vi "S2C_5190CR_Proc_Globals.vi"() -> ()   [LabVIEW 2015]
doc: "Globals for the 5190CR process."
panel:
  out "5190-Tcp":refnum<k5>
  out "5190-Refs":string[][](array[string])
  in  "5190-VI":refnum<vi>
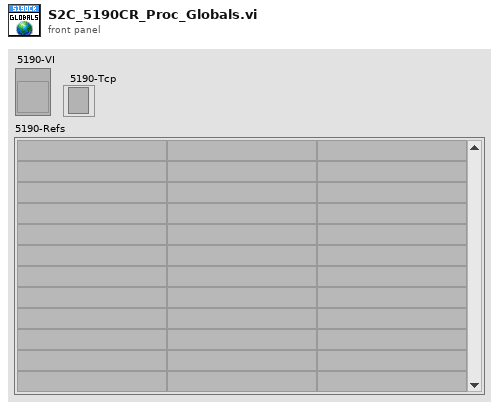
[diagram p1: front panel]
diagram:
